vi "conditional_iterate.vi"(4 "iterate?":bool, 5 "number in":u16) -> (1 "number out":u16)   [LabVIEW 2010]
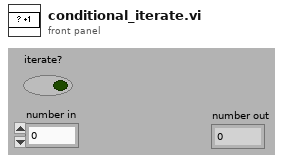
[diagram p1: front panel]
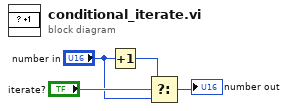
[diagram p0: block diagram]
diagram:
  n1 = Increment(x="number in") -> (x+1=w2:u16)
  n2 = Select(t=w2, s="iterate?", f="number in") -> (s? t:f=→"number out":u16)
